vi "A Switch V.5.0.vi"(8 "Input Button":bool, 11 "TIme until Reset":i32) -> (2 "On?":bool)   [LabVIEW 2016]
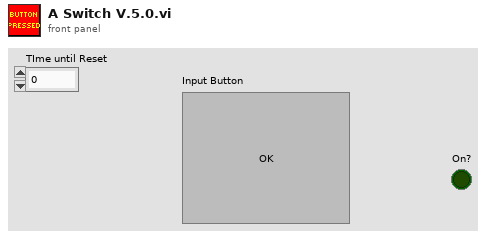
[diagram p1: front panel]
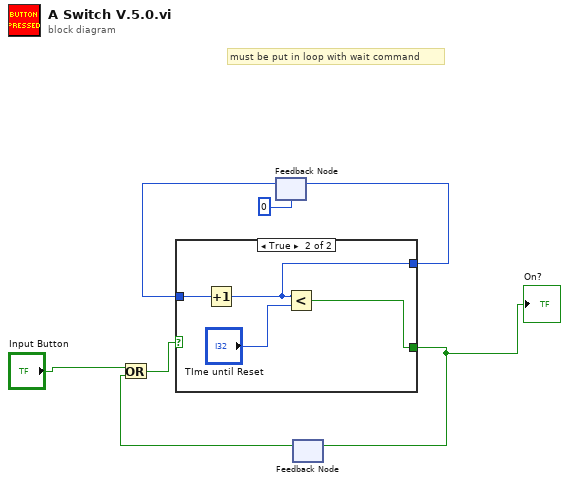
[diagram p0: block diagram]
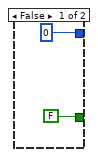
[diagram p2: hidden frame]
diagram:
  # "must be put in loop with wait command"
  n1 = feedback #1(0) -> (w6:i32)
  n2 = feedback #2() -> (w2:bool)  [unwired: 1 in]
  n3 = Or(x="Input Button", y=w2) -> (x .or. y?=w3:bool)
  n4 = case shown="True" w3 {
    tunnel: [FALSE w12] -> w4
    tunnel: w6 -> [_ w13]
    tunnel: [0 w11] -> w5
    frame False {
    }
    frame True {
      n5 = Increment(x=w13) -> (x+1=w11:i32)
      n6 = Less?(x=w11, y="TIme until Reset") -> (x < y?=w12:bool)
    }
  }
  "On?" <- w4
  n7 = feedback-in #1(w5) -> ()
  n8 = feedback-in #2(w4) -> ()
